vi "SVL Limit Testing.vi"   [LabVIEW 2017, in "SoundVib_LimitTest.lvlib"]
doc: "Performs limit testing on waveforms, spectra, XY data, identified peaks, or scalar measurements. You can specify an upper and lower boundary of the envelope to define a pass range. This VI uses the defined pass range to test the input signal. VI outputs apply only to the current input signal. You can wire output values to a graph to view the limits, signal, and failures. Wire data to the<B> signal in</B> input to determine the polymorphic instance to use or manually select the instance."
uses:
  <vilib>/addons/Sound and Vibration/svt_Limit Test/SoundVib_LimitTest.lvlib
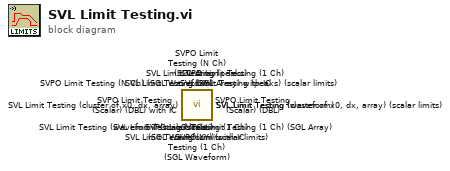
[diagram p0: block diagram]
diagram:
  n1 = call <vilib>:"SVPO Limit Testing (1 Ch) (SGL Waveform) with IC.vi"() -> ()  [unwired: 7 in, 5 out]
  n2 = call <vilib>:"SVPO Limit Testing (1 Ch) (SGL Array) with IC.vi"() -> ()  [unwired: 8 in, 4 out]
  n3 = call <vilib>:"SVPO Limit Testing (Scalar) (DBL) with IC.vi"() -> ()  [unwired: 8 in, 4 out]
  n4 = call <vilib>:"SVPO Limit Testing (Scalar) (DBL).vi"() -> ()  [unwired: 9 in, 3 out]
  n5 = call <vilib>:"SVPO Limit Testing (N Ch) (SGL Waveform).vi"() -> ()  [unwired: 8 in, 4 out]
  n6 = call <vilib>:"SVPO Limit Testing (N Ch) (SGL Array).vi"() -> ()  [unwired: 9 in, 3 out]
  n7 = call <vilib>:"SVPO Limit Testing (1 Ch) (SGL Waveform).vi"() -> ()  [unwired: 8 in, 4 out]
  n8 = call <vilib>:"SVPO Limit Testing (1 Ch) (SGL Array).vi"() -> ()  [unwired: 9 in, 3 out]
  n9 = call <vilib>:"SVL Limit Testing (cluster of x0, dx, array) (scalar limits).vi"() -> ()  [unwired: 8 in, 4 out]
  n10 = call <vilib>:"SVL Limit Testing (cluster of x0, dx, array).vi"() -> ()  [unwired: 8 in, 4 out]
  n11 = call <vilib>:"SVL Limit Testing (scalar).vi"() -> ()  [unwired: 9 in, 3 out]
  n12 = call <vilib>:"SVL Limit Testing (peaks) (scalar limits).vi"() -> ()  [unwired: 8 in, 4 out]
  n13 = call <vilib>:"SVL Limit Testing (peaks).vi"() -> ()  [unwired: 8 in, 4 out]
  n14 = call <vilib>:"SVL Limit Testing (XY) (scalar limits).vi"() -> ()  [unwired: 8 in, 4 out]
  n15 = call <vilib>:"SVL Limit Testing (XY).vi"() -> ()  [unwired: 8 in, 4 out]
  n16 = call <vilib>:"SVL Limit Testing (waveform) (scalar limits).vi"() -> ()  [unwired: 8 in, 4 out]
  n17 = call <vilib>:"SVL Limit Testing (waveform).vi"() -> ()  [unwired: 8 in, 4 out]
